vi "Resize Data with xi-axis (NaN).vi"(0 "x-axis":dbl[](array[numeric])=[0.0, 1.0, 2.0, 3.0, 4.0, 5.0, 66.0, 7.0, 8.0, 9.0], 5 "Measure data":dbl[](array[numeric])=[0.0, 1.0, 2.0, 3.0]) -> (4 "Updated Data":dbl[](array[numeric]))   [LabVIEW 2023, in "FPT Intermodulation UI.lvlib"]
uses:
  FPT Intermodulation UI.lvlib
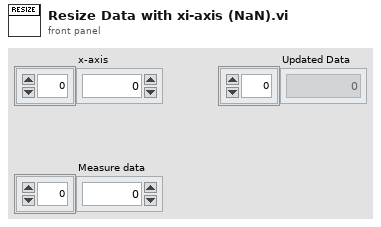
[diagram p1: front panel]
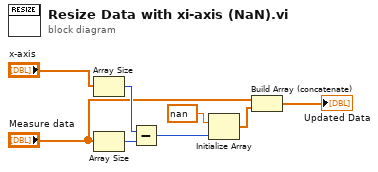
[diagram p0: block diagram]
diagram:
  n1 = Array Size(array="x-axis") -> (size(s)=w8:i32)
  n2 = Array Size(array="Measure data") -> (size(s)=w7:i32)
  n3 = Subtract(x=w8, y=w7) -> (x-y=w6:i32)
  n4 = Initialize Array(nan ("element"), w6) -> (w4:dbl[])
  n5 = Build Array (concatenate)("Measure data", w4) -> (→"Updated Data":dbl[])
